vi "QX_Read Data.vi"(8 "Error in":errorcluster, 10 "InUsedChan[]":T2, 11 "DaqMeasurement":refnum<k24>) -> (0 "Error out":errorcluster, 1 "data":dbl[][](array[numeric]), 2 "data":waveform(dbl)[](array[waveform]), 3 "DaqMeasurement":refnum<k24>)   [LabVIEW 2016]
doc: "Delivers measurement values in a standard LabVIEW format ( first timestamp of the measurement values in utc time format, the samplerate in 1/samplerate in Hz, and an array of measurement values).\n\nDaqMeasurement: Reference to the DaqMeasurement instance\nIndex: The index of the singnal within the given array of signals from which the measurement values should be delivered."
uses:
  Ctrls/HardWare _ Channel Parameters.ctl
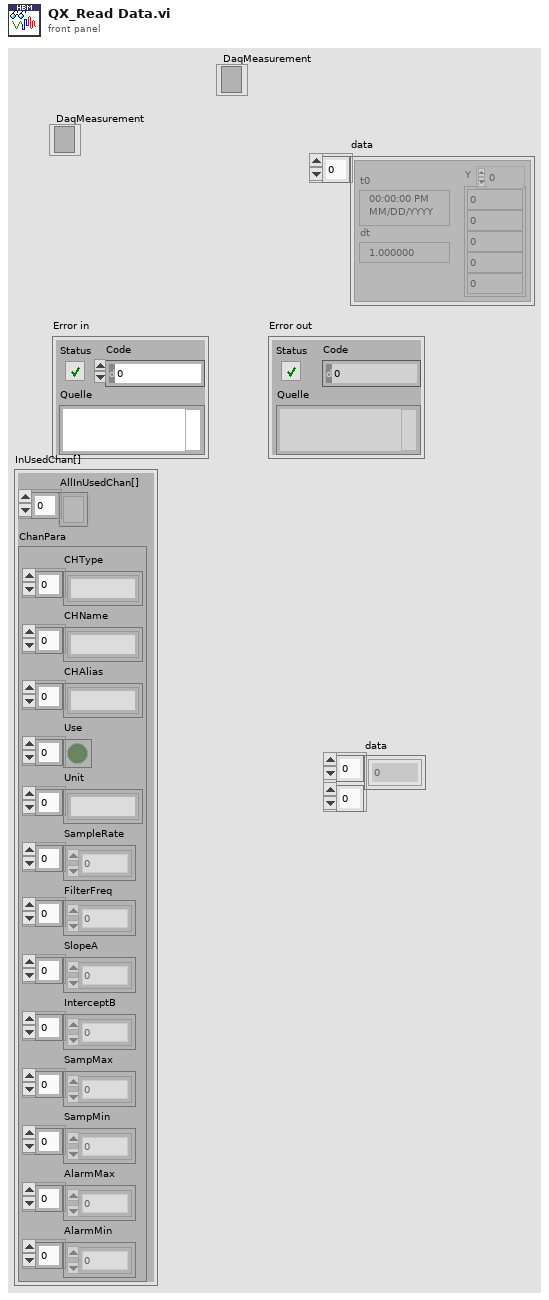
[diagram p1: front panel]
types:
  T1 = typedef "HardWare _ Channel Parameters.ctl" = cluster{"CHType":string[], "CHName":string[], "CHAlias":string[], "Use":bool[], "Unit":string[], "SampleRate":dbl[], "FilterFreq":dbl[], "SlopeA":dbl[], "InterceptB":dbl[], "SampMax":dbl[], "SampMin":dbl[], "AlarmMax":dbl[], "AlarmMin":dbl[]}
  T2 = cluster{"AllInUsedChan[]":refnum<k24>[], "ChanPara":T1}
  T3 = typedef "LVDateTimeRec.ctl" = cluster{"Sekundenbruchteil":dbl, "Sekunde":i32, "Minute":i32, "Stunde":i32, "Tag des Monats":i32, "Monat":i32, "Jahr":i32, "Wochentag":i32, "Tag des Jahres":i32, "DST":i32}
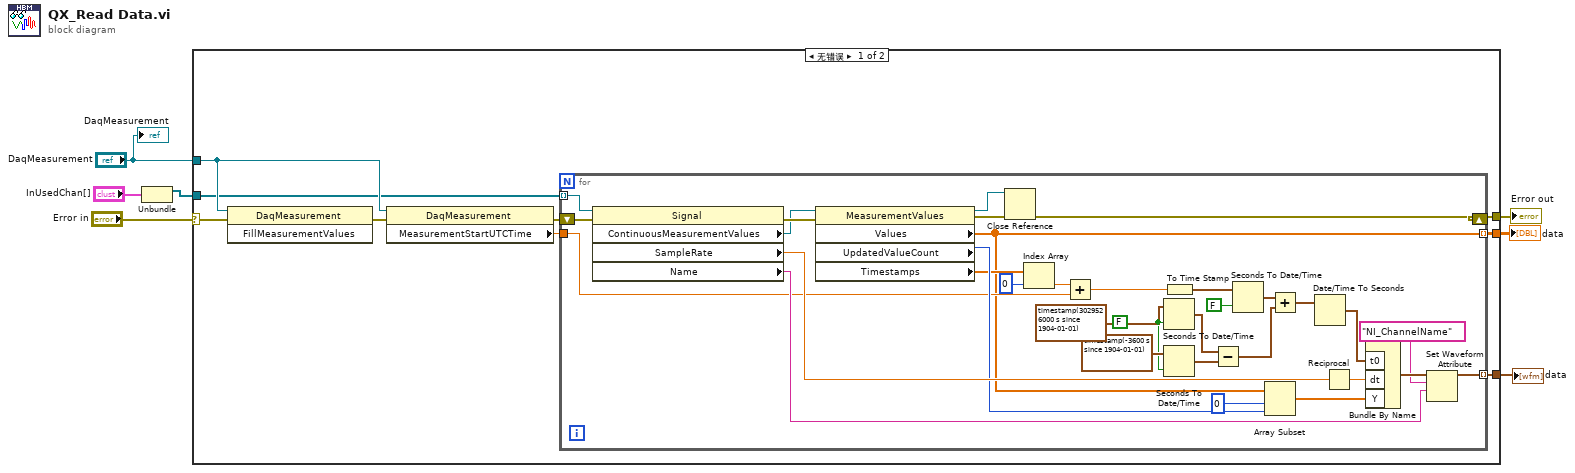
[diagram p0: block diagram]
diagram:
  n1 = Unbundle("InUsedChan[]") -> ("AllInUsedChan[]"=w2:refnum<k24>[])  [unwired: 1 out]
  n2 = case shown="无错误" "Error in" {
    selector: "Error in" -> [w13 w50]
    tunnel: "DaqMeasurement" -> [w11 _]
    tunnel: w2 -> [w10 _]
    tunnel: [w14 w50] -> w6
    tunnel: [w15 _] -> w5
    tunnel: [w8 _] -> w1
    frame No Error {
      n3 = invoke on="Methodenknoten" class="DaqMeasurement" method="FillMeasurementValues"(reference=w11, error in=w13) -> (error out=w12:errorcluster)  [unwired: 1 in, 2 out]
      n4 = property on="Eigenschaftsknoten" class="DaqMeasurement"(reference=w11, error in=w12) -> (error out=w16:errorcluster, "MeasurementStartUTCTime"=w9:dbl)  [unwired: 1 out]
      n5 = for {
        tunnel: [w27] -> w15 mode=indexing
        shift-right: [w22] -> w14
        shift-left: w16 -> [w29]
        tunnel: w10 -> [w20] mode=indexing
        tunnel: w9 -> [w19]
        tunnel: [w17] -> w8 mode=indexing
        w38 = FALSE ("in Weltzeit (F)")
        n6 = property on="Eigenschaftsknoten" class="Signal"(reference=w20, error in=w29) -> (error out=w49:errorcluster, "ContinuousMeasurementValues"=w23:refnum<k24>, "SampleRate"=w47:dbl, "Name"=w26:string)  [unwired: 1 out]
        n7 = property on="Eigenschaftsknoten" class="MeasurementValues"(reference=w23, error in=w49) -> (reference out=w21:refnum<k24>, error out=w24:errorcluster, "Values"=w17:dbl[], "UpdatedValueCount"=w44:i32, "Timestamps"=w18:dbl[])
        n8 = Close Reference(reference=w21, error in (no error)=w24) -> (error out=w22:errorcluster)
        n9 = Index Array(array=w18, index=0 ("Index")) -> (element=w42:dbl)
        n10 = Add(x=w42, y=w19) -> (x+y=w41:dbl)
        n11 = Seconds To Date/Time(time stamp (now)=timestamp(3029526000 s since 1904-01-01), to UTC (F)=w38) -> (date time rec=w30:T3)
        n12 = Seconds To Date/Time(time stamp (now)=timestamp(-3600 s since 1904-01-01), to UTC (F)=w38) -> (date time rec=w31:T3)
        n13 = To Time Stamp(1:w41) -> (0:w37:timestamp)
        n14 = Subtract(x=w30, y=w31) -> (x-y=w35:T3)
        n15 = Seconds To Date/Time(time stamp (now)=w37, to UTC (F)=FALSE ("in Weltzeit (F)")) -> (date time rec=w36:T3)
        n16 = Array Subset(array=w17, index=0 ("Index"), length=w44) -> (w43:dbl[])
        n17 = Add(x=w36, y=w35) -> (x+y=w34:T3)
        n18 = Date/Time To Seconds(2:w34) -> (0:w33:timestamp)  [unwired: 1 in]
        n19 = Reciprocal(x=w47) -> (1/x=w46:dbl)
        n20 = Bundle By Name("t0"=w33, "dt"=w46, "Y"=w43) -> (w28:waveform(dbl))  [unwired: 1 in]
        n21 = Set Waveform Attribute(5:w26, 6:"NI_ChannelName" ("Channel Name"), 7:w28) -> (3:w27:waveform(dbl))  [unwired: 1 in, 2 out]
      }
    }
    frame Error {
    }
  }
  "Error out" <- w6
  "data" <- w5
  "data" <- w1
  "DaqMeasurement" <- "DaqMeasurement"
